vi "Coerce Format String.vi"(1 "Format String":string) -> (0 "Coerced String":string)   [LabVIEW 2018, in "Numeric Data Type.lvclass"]
uses:
  Numeric Data Type.lvclass
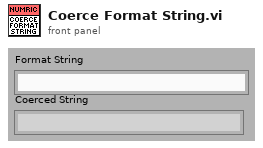
[diagram p1: front panel]
types:
  T1 = typedef "Numeric Data Type.lvclass/Time Info.ctl" = cluster{"Time Format":T2, "Numeric Format":T3, "Clock Type":T4, "Include Seconds?":bool, "Seconds Precision":i16, "Date Order":T5, "Date Format":T6, "Year Format":T7, "UTC":i16}
  T2 = typedef "Numeric Data Type.lvclass/Time Format.ctl" = enum16{"Custom time format", "System time format", "Time unused"}
  T3 = typedef "Numeric Data Type.lvclass/Numeric Format Enum.ctl" = enum16{"Floating Point Notation", "Scientific Notation", "Engineering Notation", "SI Notation", "<not used>", "Decimal", "Hexadecimal", "Octal", "Binary", "<not used 2>", "Absolute Time", "Relative Time"}
  T4 = typedef "Numeric Data Type.lvclass/Clock Type.ctl" = enum32{"12-Hour (AM/PM)", "24-Hour"}
  T5 = typedef "Numeric Data Type.lvclass/Date Order.ctl" = enum32{"M/D/Y", "D/M/Y", "Y/M/D"}
  T6 = typedef "Numeric Data Type.lvclass/Date Format.ctl" = enum16{"Custom date format", "System date format", "Date unused"}
  T7 = typedef "Numeric Data Type.lvclass/Year Format.ctl" = enum32{"No Year", "2-digit Year", "4-digit Year"}
  T8 = typedef "Numeric Data Type.lvclass/Numeric Info.ctl" = cluster{"Minimum Field Width":i32, "Digits of Precision":i32, "Numeric Format":T3, "Precision Type":T9, "Hide trailing zeros":bool, "exponent":bool, "just/pad":T10, "Modifiers":string}
  T9 = typedef "Numeric Data Type.lvclass/Precision Type.ctl" = enum16{"Digits of precision", "Significant digits"}
  T10 = typedef "Numeric Data Type.lvclass/Padding.ctl" = enum16{"Pad with spaces on left", "Pad with spaces on right", "Pad with zeros on left"}
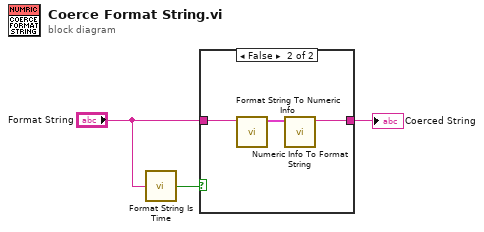
[diagram p0: block diagram]
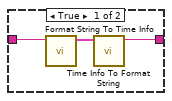
[diagram p2: hidden frame]
diagram:
  n1 = call "Format String Is Time.vi"("Format String"="Format String") -> ("Time?"=w1:bool)
  n2 = case shown="False" w1 {
    tunnel: "Format String" -> [w6 w9]
    tunnel: [w4 w7] -> w3
    frame True {
      n3 = call "Format String To Time Info.vi"("Format String"=w6) -> ("Time Info"=w5:T1)  [unwired: 10 in]
      n4 = call "Time Info To Format String.vi"("Time Format & Precision Info"=w5) -> ("Format String"=w4:string)  [unwired: 10 in]
    }
    frame False {
      n5 = call "Format String To Numeric Info.vi"("Format String"=w9) -> ("Numeric Format & Precision Info"=w8:T8)  [unwired: 10 in]
      n6 = call "Numeric Info To Format String.vi"("Numeric Format & Precision Info"=w8) -> ("Format String"=w7:string)  [unwired: 10 in]
    }
  }
  "Coerced String" <- w3
